vi "SerialNumber to DeviceName.vi"(9 "NI2 Serial Number":dbl, 10 "NI1 Serial Number":dbl) -> (1 "NI2 Device Name":tag, 2 "NI1 Device Name":tag)   [LabVIEW 2017]
uses:
  <resource>/objmgr/daqmx.rc
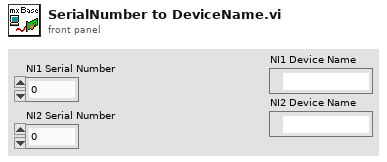
[diagram p1: front panel]
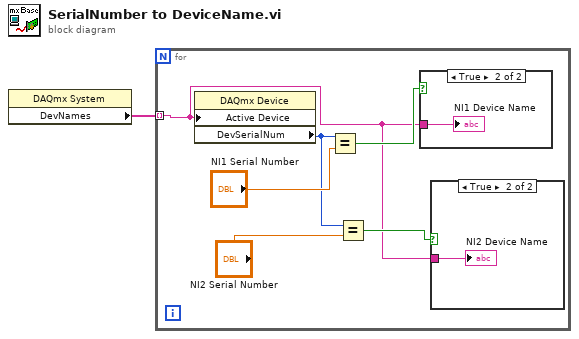
[diagram p0: block diagram]
diagram:
  n1 = property class="DAQmx System"() -> ("DevNames"=w1:tag[])  [unwired: 2 in, 2 out]
  n2 = for {
    tunnel: w1 -> [w2] mode=indexing
    n3 = property class="DAQmx Device"("Active Device"=w2) -> ("DevSerialNum"=w5:u32)  [unwired: 2 in, 2 out]
    n4 = Equal?(x=w5, y="NI1 Serial Number") -> (x = y?=w6:bool)
    n5 = Equal?(x=w5, y="NI2 Serial Number") -> (x = y?=w3:bool)
    n6 = case shown="True" w6 {
      tunnel: w2 -> [_ w9]
      frame False {
      }
      frame True {
        "NI1 Device Name" <- w9
      }
    }
    n7 = case shown="True" w3 {
      tunnel: w2 -> [_ w8]
      frame False {
      }
      frame True {
        "NI2 Device Name" <- w8
      }
    }
  }
